vi "Script Parse Project Modules Constants.vi"(7 "App Ref":refnum<vi>, 8 "error in":errorcluster, 11 "All DQMH Modules Refs":refnum<vi>[](array[refnum])) -> (0 "error out":errorcluster, 3 "Project Info Results":T1[](array[typedef]))   [LabVIEW 2019, in "Panther Dashboard.lvlib"]
uses:
  Panther Dashboard.lvlib
  Module Info--cluster.ctl
  <vilib>/Utility/traverseref.llb/TRef TravTarget.ctl
  <vilib>/Utility/traverseref.llb/VI Scripting - Traverse.lvlib
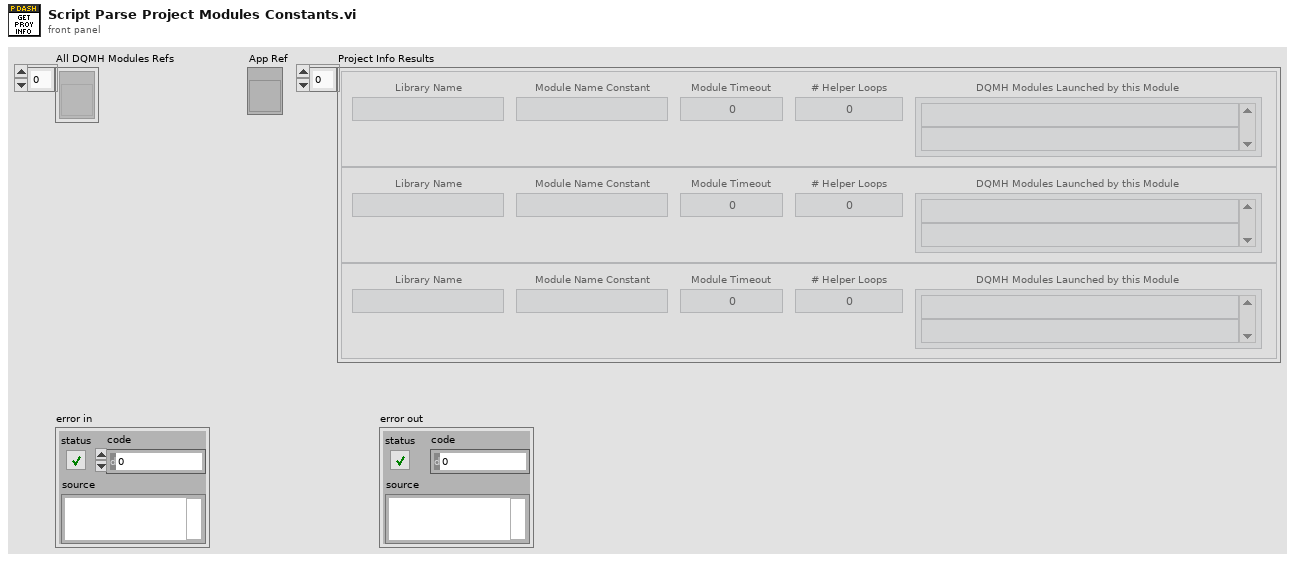
[diagram p1: front panel]
types:
  T1 = typedef "Panther Dashboard.lvlib/Module Info--cluster.ctl" = cluster{"Library Name":string, "Module Name Constant":string, "Module Timeout":i32, "# Helper Loops":i32, "DQMH Modules Launched by this Module":string[]}
  T2 = typedef "TRef TravTarget.ctl" = enum16{"FP", "BD", "Other"}
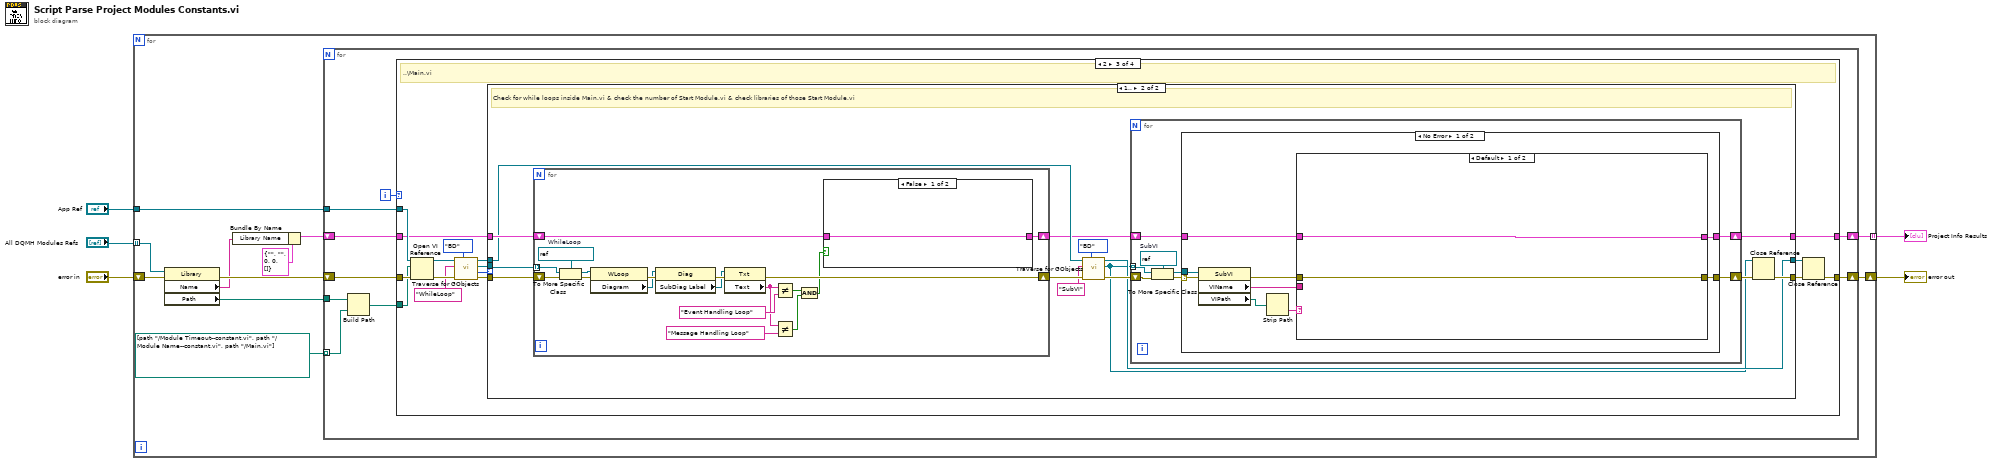
[diagram p0: block diagram]
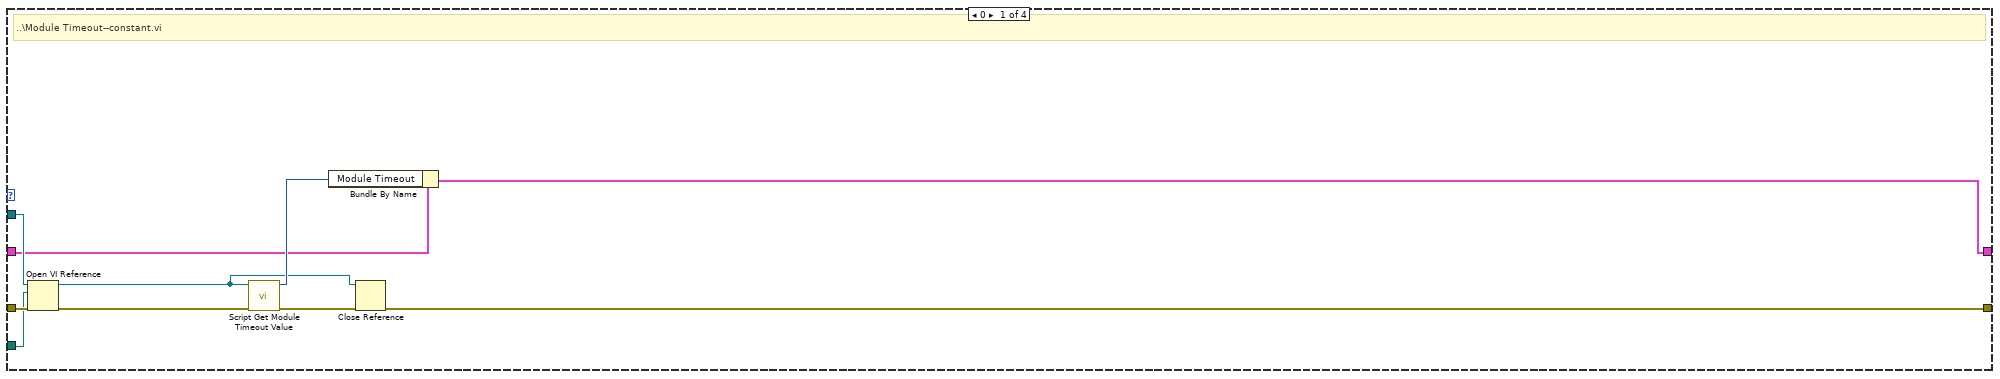
[diagram p2: hidden frame]
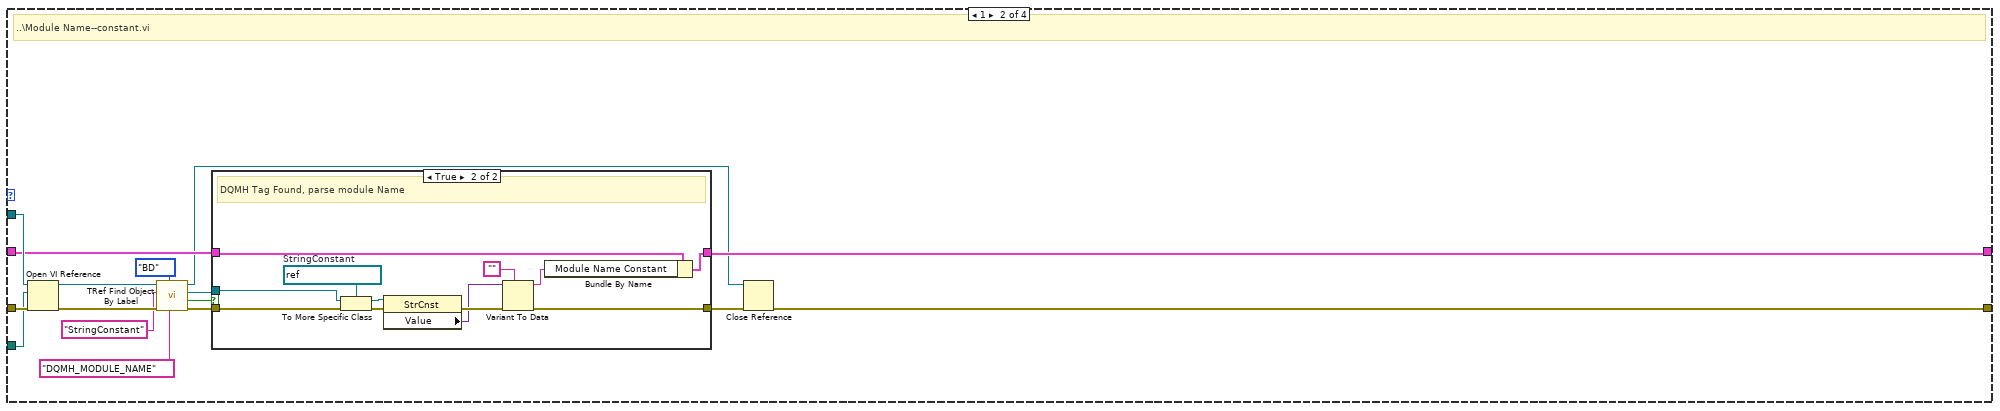
[diagram p3: hidden frame]
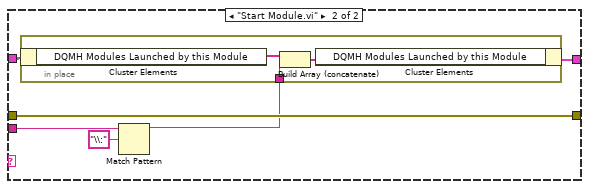
[diagram p6: hidden frame]
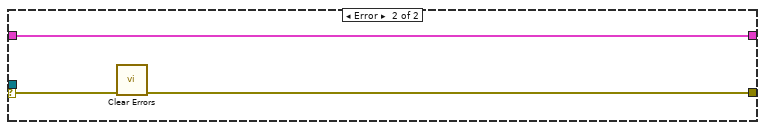
[diagram p7: hidden frame]
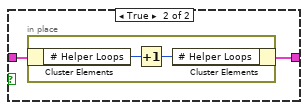
[diagram p8: hidden frame]
diagram:
  n1 = for {
    tunnel: "All DQMH Modules Refs" -> [w12] mode=indexing
    tunnel: "App Ref" -> [w11]
    shift-right: [w14] -> w4
    shift-left: "error in" -> [w15]
    tunnel: [w9] -> w1 mode=indexing
    n2 = property class="Library"(reference=w12, error in=w15) -> (error out=w16:errorcluster, "Name"=w6:string, "Path"=w7:path)  [unwired: 1 out]
    n3 = Bundle By Name(cluster=T1 {"Library Name"="", "Module Name Constant"="", "Module Timeout"=0, "# Helper Loops"=0, "DQMH Modules Launched by this Module"=[]} ("Module Specifics"), "Library Name"=w6) -> (w8:T1)
    n4 = for {
      tunnel: w7 -> [w23]
      tunnel: path[] [path "../Module Timeout--constant.vi", path "../Module Name--constant.vi", path "../Main.vi"] -> [w22] mode=indexing
      shift-right: [w24] -> w14
      shift-left: w16 -> [w25]
      tunnel: w11 -> [w19]
      shift-right: [w18] -> w9
      shift-left: w8 -> [w17]
      i -> [w20]
      n5 = Build Path(base path=w23, name or relative path=w22) -> (appended path=w21:path)
      n6 = case shown="2" w20 {
        tunnel: w21 -> [w32 w41 w72 _]
        tunnel: w25 -> [w34 w49 w79 w154]
        tunnel: w19 -> [w31 w39 w70 _]
        tunnel: [w27 w47 w77 w154] -> w24
        tunnel: [w29 w38 w69 w153] -> w18
        tunnel: w17 -> [w28 w37 w68 w153]
        frame 0 {
          # "..\\Module Timeout--constant.vi"
          n7 = Open VI Reference(application reference (local)=w31, vi path=w32, error in (no error)=w34) -> (vi reference=w26:refnum<vi>, error out=w35:errorcluster)  [unwired: 3 in]
          n8 = call "Script Get Module Timeout Value.vi"("error in"=w35, "VI in"=w26) -> ("error out"=w33:errorcluster, "Module Timeout"=w30:i32)  [unwired: 8 in]
          n9 = Bundle By Name(cluster=w28, "Module Timeout"=w30) -> (w29:T1)
          n10 = Close Reference(reference=w26, error in (no error)=w33) -> (error out=w27:errorcluster)
        }
        frame 1 {
          # "..\\Module Name--constant.vi"
          n11 = Open VI Reference(application reference (local)=w39, vi path=w41, error in (no error)=w49) -> (vi reference=w40:refnum<vi>, error out=w48:errorcluster)  [unwired: 3 in]
          n12 = call <vilib>:"TRef Find Object By Label.vi"("Label"="DQMH_MODULE_NAME", "Traverse Target"=TRef_TravTarget."BD", "error in (no error)"=w48, "Class Name"="StringConstant", "VI Ref"=w40) -> ("error out"=w51:errorcluster, "Found?"=w43:bool, "Found Obj Ref"=w44:refnum<vi>, "dup VI Ref"=w36:refnum<vi>)  [unwired: 3 in]
          n13 = case shown="True" w43 {
            tunnel: w51 -> [w53 w65]
            tunnel: w44 -> [_ w61]
            tunnel: [w53 w62] -> w50
            tunnel: [w52 w55] -> w38
            tunnel: w37 -> [w52 w54]
            frame False {
            }
            frame True {
              w60 = refnum<vi> refnum  # StringConstant
              # "DQMH Tag Found, parse module Name"
              n14 = To More Specific Class(target class=w60, reference=w61, error in=w65) -> (specific class reference=w59:refnum<vi>, error out=w64:errorcluster)
              n15 = property class="StrCnst"(reference=w59, error in=w64) -> (error out=w63:errorcluster, "Value"=w58:variant)  [unwired: 1 out]
              n16 = Variant To Data(error in=w63, type="", Variant=w58) -> (data=w56:string, error out=w62:errorcluster)
              n17 = Bundle By Name(cluster=w54, "Module Name Constant"=w56) -> (w55:T1)
            }
          }
          n18 = Close Reference(reference=w36, error in (no error)=w50) -> (error out=w47:errorcluster)
        }
        frame 2 {
          # "..\\Main.vi"
          n19 = Open VI Reference(application reference (local)=w70, vi path=w72, error in (no error)=w79) -> (vi reference=w71:refnum<vi>, error out=w78:errorcluster)  [unwired: 3 in]
          n20 = call <vilib>:"Traverse for GObjects.vi"("Traverse Target"=TRef_TravTarget."BD", "error in (no error)"=w78, "Class Name"="WhileLoop", "VI Refnum"=w71) -> ("error out"=w81:errorcluster, "# of Refs"=w66:i32, "References"=w75:refnum<vi>[], "dup VI Refnum"=w74:refnum<vi>)  [unwired: 4 in]
          n21 = case shown="1.." w66 {
            tunnel: w81 -> [w84 w98]
            tunnel: w75 -> [_ w93]
            tunnel: w74 -> [w83 w91]
            tunnel: [w83 w90] -> w73
            tunnel: [w84 w94] -> w80
            tunnel: [w82 w86] -> w69
            tunnel: w68 -> [w82 w92]
            frame 0, Default {
            }
            frame 1.. {
              # "Check for while loops inside Main.vi & check the number of Start Module.vi & check libraries of those Start Module.vi"
              n22 = for {
                tunnel: w93 -> [w142] mode=indexing
                shift-right: [w143] -> w97
                shift-left: w98 -> [w147]
                shift-right: [w131] -> w87
                shift-left: w92 -> [w139]
                w141 = refnum<vi> refnum  # WhileLoop
                n23 = To More Specific Class(target class=w141, reference=w142, error in=w147) -> (specific class reference=w140:refnum<vi>, error out=w146:errorcluster)
                n24 = property class="WLoop"(reference=w140, error in=w146) -> (error out=w145:errorcluster, "Diagram"=w138:refnum<vi>)  [unwired: 1 out]
                n25 = property class="Diag"(reference=w138, error in=w145) -> (error out=w144:errorcluster, "SubDiag Label"=w137:refnum<vi>)  [unwired: 1 out]
                n26 = property class="Txt"(reference=w137, error in=w144) -> (error out=w143:errorcluster, "Text"=w130:string)  [unwired: 1 out]
                n27 = Not Equal?(x=w130, y="Event Handling Loop") -> (x != y?=w135:bool)
                n28 = Not Equal?(x=w130, y="Message Handling Loop") -> (x != y?=w133:bool)
                n29 = And(x=w135, y=w133) -> (x .and. y?=w132:bool)
                n30 = case shown="False" w132 {
                  tunnel: w139 -> [w148 w150]
                  tunnel: [w148 w149] -> w131
                  frame False {
                  }
                  frame True {
                    n31 = in-place {
                      n32 = in-place-cluster #1(w150) -> ("# Helper Loops"=w152:i32)
                      n33 = Increment(x=w152) -> (x+1=w151:i32)
                      n34 = in-place-cluster #1("# Helper Loops"=w151) -> (w149:T1)
                    }
                  }
                }
              }
              n35 = call <vilib>:"Traverse for GObjects.vi"("Traverse Target"=TRef_TravTarget."BD", "error in (no error)"=w97, "Class Name"="SubVI", "VI Refnum"=w91) -> ("error out"=w96:errorcluster, "References"=w85:refnum<vi>[], "dup VI Refnum"=w90:refnum<vi>)  [unwired: 4 in, 1 out]
              n36 = for {
                tunnel: w85 -> [w103] mode=indexing
                shift-right: [w104] -> w95
                shift-left: w96 -> [w106]
                shift-right: [w99] -> w86
                shift-left: w87 -> [w100]
                w102 = refnum<vi> refnum  # SubVI
                n37 = To More Specific Class(target class=w102, reference=w103, error in=w106) -> (specific class reference=w101:refnum<vi>, error out=w105:errorcluster)
                n38 = case shown="No Error" w105 {
                  selector: w105 -> [w115 w129]
                  tunnel: w101 -> [w112 _]
                  tunnel: [w113 w128] -> w104
                  tunnel: w100 -> [w111 w127]
                  tunnel: [w110 w127] -> w99
                  frame No Error {
                    n39 = property class="SubVI"(reference=w112, error in=w115) -> (error out=w114:errorcluster, "VIName"=w108:string, "VIPath"=w107:path)  [unwired: 1 out]
                    n40 = Strip Path(path=w107) -> (name=w109:string)  [unwired: 1 out]
                    n41 = case shown="Default" w109 {
                      tunnel: w111 -> [w116 w122]
                      tunnel: w114 -> [w117 w123]
                      tunnel: [w117 w123] -> w113
                      tunnel: [w116 w121] -> w110
                      tunnel: w108 -> [_ w120]
                      frame Default {
                      }
                      frame "Start Module.vi" {
                        n42 = Match Pattern(string=w120, regular expression="\\:") -> (before substring=w118:string)  [unwired: 1 in, 3 out]
                        n43 = in-place {
                          in-place-border: w118 -> [w124]
                          n44 = in-place-cluster #2(w122) -> ("DQMH Modules Launched by this Module"=w126:string[])
                          n45 = Build Array (concatenate)(w126, w124) -> (w125:string[])
                          n46 = in-place-cluster #2("DQMH Modules Launched by this Module"=w125) -> (w121:T1)
                        }
                      }
                    }
                  }
                  frame Error {
                    n47 = call <vilib>:"Clear Errors.vi"("error in (no error)"=w129) -> ("error out"=w128:errorcluster)  [unwired: 5 in, 1 out]
                  }
                }
              }
              n48 = Close Reference(reference=w85, error in (no error)=w95) -> (error out=w94:errorcluster)
            }
          }
          n49 = Close Reference(reference=w73, error in (no error)=w80) -> (error out=w77:errorcluster)
        }
        frame Default {
        }
      }
    }
  }
  "error out" <- w4
  "Project Info Results" <- w1
